vi "Tusk.KillMessageCore.vi"(8 "error in (no error)":errorcluster, 10 "Message":refnum<class "Message.lvclass">, 11 "Tusk in":refnum<class "Tusk.lvclass">) -> (0 "error out":errorcluster, 3 "Tusk out":refnum<class "Tusk.lvclass">)   [LabVIEW 2018, in "Application.lvlib" / "Tusk.lvclass"]
uses:
  Tusk.lvclass
  Message Class/Message.lvclass
  Tusk.lvclass/Tusk.ctl
  <vilib>/event_ctls.llb/usereventprio.ctl
  Exceptions Class/Exceptions.lvclass
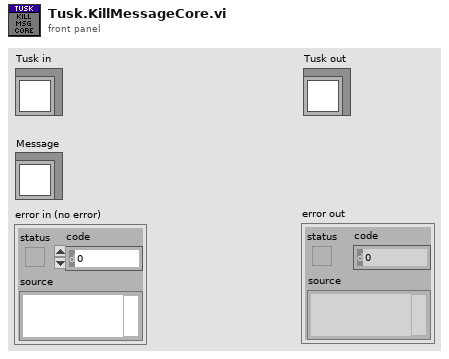
[diagram p1: front panel]
types:
  T1 = typedef "Type.ctl" = enum16{"None", "Queue", "Event", "Notifier"}
  T2 = typedef "Application.lvlib/Message.lvclass/Event Registration Refnum.ctl" = refnum<event-registration>
  T3 = typedef "usereventprio.ctl" = enum32{"high priority", "normal priority"}
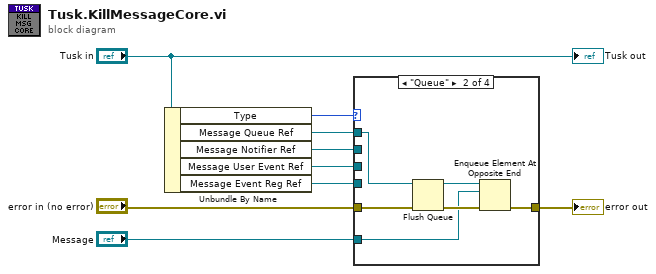
[diagram p0: block diagram]
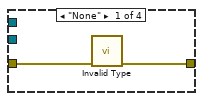
[diagram p2: hidden frame]
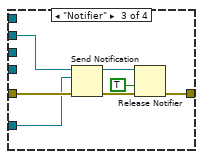
[diagram p3: hidden frame]
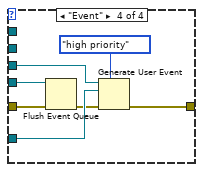
[diagram p4: hidden frame]
diagram:
  n1 = Unbundle By Name("Tusk in") -> ("Type"=w8:T1, "Message Queue Ref"=w7:refnum<queue>, "Message Notifier Ref"=w6:refnum<notifier>, "Message User Event Ref"=w5:refnum<user-event>, "Message Event Reg Ref"=w1:T2)
  n2 = case shown="\"Queue\"" w8 {
    tunnel: w7 -> [_ w15 _ _]
    tunnel: w6 -> [_ _ w23 _]
    tunnel: w5 -> [_ _ _ w31]
    tunnel: "error in (no error)" -> [w11 w16 w24 w28]
    tunnel: [w10 w17 w19 w29] -> w2
    tunnel: "Message" -> [_ w12 w22 w30]
    tunnel: w1 -> [_ _ _ w27]
    frame "None" {
      n3 = call "Invalid Type.vi"("error in (no error)"=w11) -> ("error out"=w10:errorcluster)  [unwired: 10 in]
    }
    frame "Queue" {
      n4 = Flush Queue(queue=w15, error in (no error)=w16) -> (queue out=w14:refnum<queue>, error out=w13:errorcluster)  [unwired: 1 out]
      n5 = Enqueue Element At Opposite End(queue=w14, element=w12, error in (no error)=w13) -> (error out=w17:errorcluster)  [unwired: 1 in, 2 out]
    }
    frame "Notifier" {
      n6 = Send Notification(notification=w22, notifier=w23, error in (no error)=w24) -> (notifier out=w20:refnum<notifier>, error out=w21:errorcluster)
      n7 = Release Notifier(notifier=w20, force destroy? (F)=TRUE, error in (no error)=w21) -> (error out=w19:errorcluster)  [unwired: 2 out]
    }
    frame "Event" {
      n8 = Flush Event Queue(0:w27, 3:w28) -> (11:w26:errorcluster)  [unwired: 4 in, 2 out]
      n9 = Generate User Event(priority (normal)=usereventprio."high priority", user event=w31, event data cluster=w30, error in=w26) -> (error out=w29:errorcluster)  [unwired: 1 out]
    }
  }
  "error out" <- w2
  "Tusk out" <- "Tusk in"
